vi "GagePeakHisto.vi"() -> ()   [LabVIEW 2017]
uses:
  <vilib>/measure/mamon.llb/Waveform Peak Detection for N Chan.vi
  <vilib>/Waveform/WDTOps.llb/WDT Append Waveforms DBL.vi
  <instrlib>/niHWS/nihws.llb/niHWS Store Analog Waveform DBL.vi
  <vilib>/measure/NI_MAPro.lvlib
panel:
  in  "Save waveform":bool
  in  "Save to:":path
  in  "Stop":bool
  out "Dead time (%)":dbl
  in  "Save to:":path
  in  "Save Peaks Hight":bool
  out "ChA: Histogram Peaks":dynamicdata(graph)
  in  "Peak threshold":dbl=0.5 format="%.2p"
  out "Board":string
  out "1st segment TS":string
  out "Time Interval Graph":cluster{i32[], dbl[]}(graph)
  out "Tick Frequency, Hz":u32
  in  "Trigger":T1={"Slope"=0, "Level (%)"=20, "Source"=0, "External Range"=2000, "External Coupling"=0, "External"=FALSE, "Disable"=FALSE, "External Impedance"=1} {"External Impedance" items=["50 Ohm", "HiZ"]; "External Coupling" items=["DC", "AC"]; "External Range" min=2000 max=10000 step=8000; "Slope" items=["Rising", "Falling"]; "Level (%)" min=-100 max=100; "Source" min=0 max=64 step=1}
  in  "Reset":bool
  in  "Counter source":bool
  out "Array":dbl[](array[numeric]) format="%.2f"
  out "Status":string
  in  "Channels":T2(array[cluster])=[{"Coupling"=0, "Differential Input"=FALSE, "Direct-to-ADC"=FALSE, "Range"=2000, "Impedance"=50, "DC Offset"=0, "Filter"=0}] {"Impedance" min=50 max=1000000 step=999950; "Coupling" items=["DC", "AC"]}
  in  "Acquisition":T3={"Sample Rate"=10000000.0, "Mode"=0, "Trigger Position\nin Record(%)"=50.0, "Record lenght(s)"=1.0, "Trigger Timeout(s)"=1000000.0, "Trigger Delay(s)"=0.0, "Clock mode"=enum."Internal", "Number Of Records"=10} {"Record lenght(s)" min=1.6e-05 step=1e-06 format="%.0p"; "Trigger Delay(s)" min=0.0 step=1e-06 format="%.0p"; "Trigger Position\nin Record(%)" min=0.0 step=1.0; "Mode" items=["Single", "Dual", "Quad", "Octal"]; "Sample Rate" format="%.0p"}
  in  "Length":dbl=512.0 min=0.0 step=1.0
  in  "Start Point":dbl
  out "Waveform Graph":cluster{dbl, dbl, "Data in Volts":dbl[][]}(graph) caption="Record 8  of  10"
  # "Number of records"
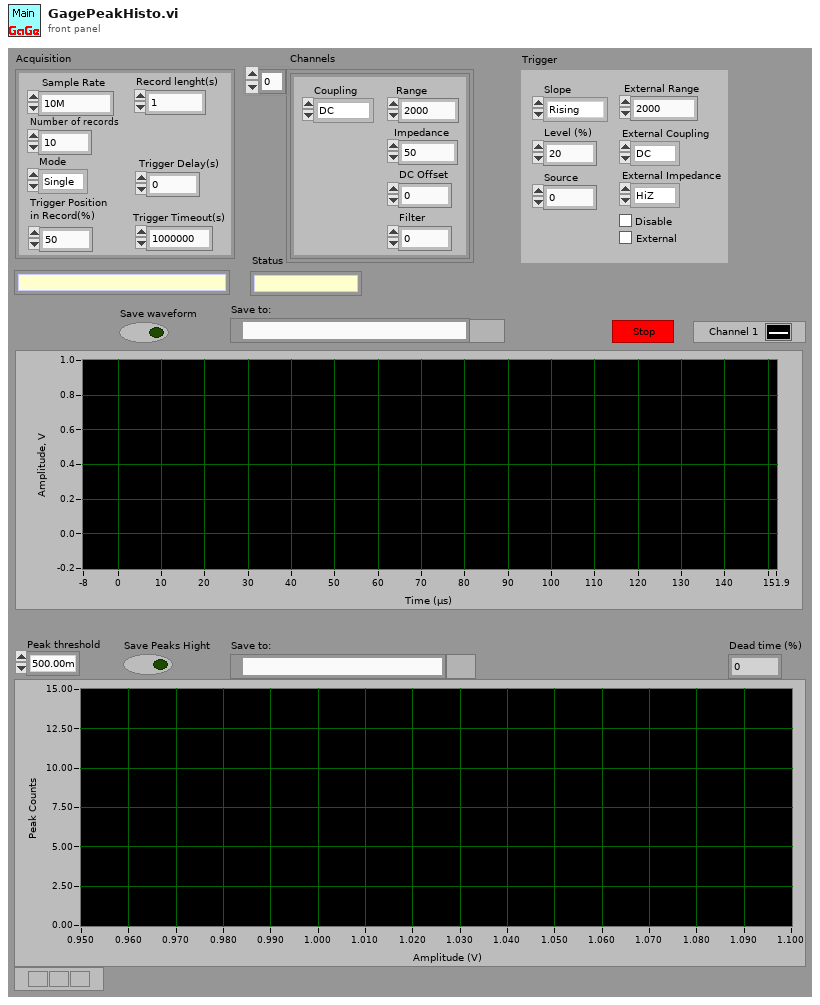
[diagram p1: front panel]
types:
  T1 = cluster{"Slope":u16, "Level (%)":i32, "Source":i32, "External Range":u32, "External Coupling":u16, "External":bool, "Disable":bool, "External Impedance":u16}
  T2 = cluster{"Coupling":u16, "Differential Input":bool, "Direct-to-ADC":bool, "Range":u32, "Impedance":u32, "DC Offset":i32, "Filter":i32}[]
  T3 = cluster{"Sample Rate":dbl, "Mode":u16, "Trigger Position\nin Record(%)":dbl, "Record lenght(s)":dbl, "Trigger Timeout(s)":dbl, "Trigger Delay(s)":dbl, "Clock mode":enum16{"Internal", "External", "Reference"}, "Number Of Records":u32}
  T4 = enum16{"big-endian, network order", "native, host order", "little-endian"}
  T5 = cluster{"Handle":u32, "Sample size":u32, "Resolution":i32, "Offset":i32, "Channels":u32, "Boards":u32}
  T6 = cluster{"Coupling":u16, "Differential Input":bool, "Direct-to-ADC":bool, "Range":u32, "Impedance":u32, "DC Offset":i32, "Filter":i32}
  T7 = cluster{string, "Differential Input":bool, "Direct-to-ADC":bool, "Range":u32, "Impedance":u32, "DC Offset":i32, u32}
  T8 = cluster{"RingText.Text":string, "Level (%)":i32, "Source":i32, "External Range":u32, "RingText.Text":string, "External":bool, "Disable":bool, "RingText.Text":string}
  T9 = cluster{"RingText.Text":string, "Level (%)":i32, "Source":i32, "External Range":u32, "RingText.Text":string, "External":bool, "Disable":bool, "RingText.Text":string}[]
  T10 = cluster{"Sample Rate":dbl, "Clock mode":enum16{"Internal", "External", "Reference"}, "RingText.Text":string, dbl, dbl, dbl, dbl, "Trigger Delay(s)":dbl}
  T11 = cluster{"Handle":u32, "Sample Size":u32, "Resolution":i32, "Offset":i32, "Channels":u32, "Boards":u32}
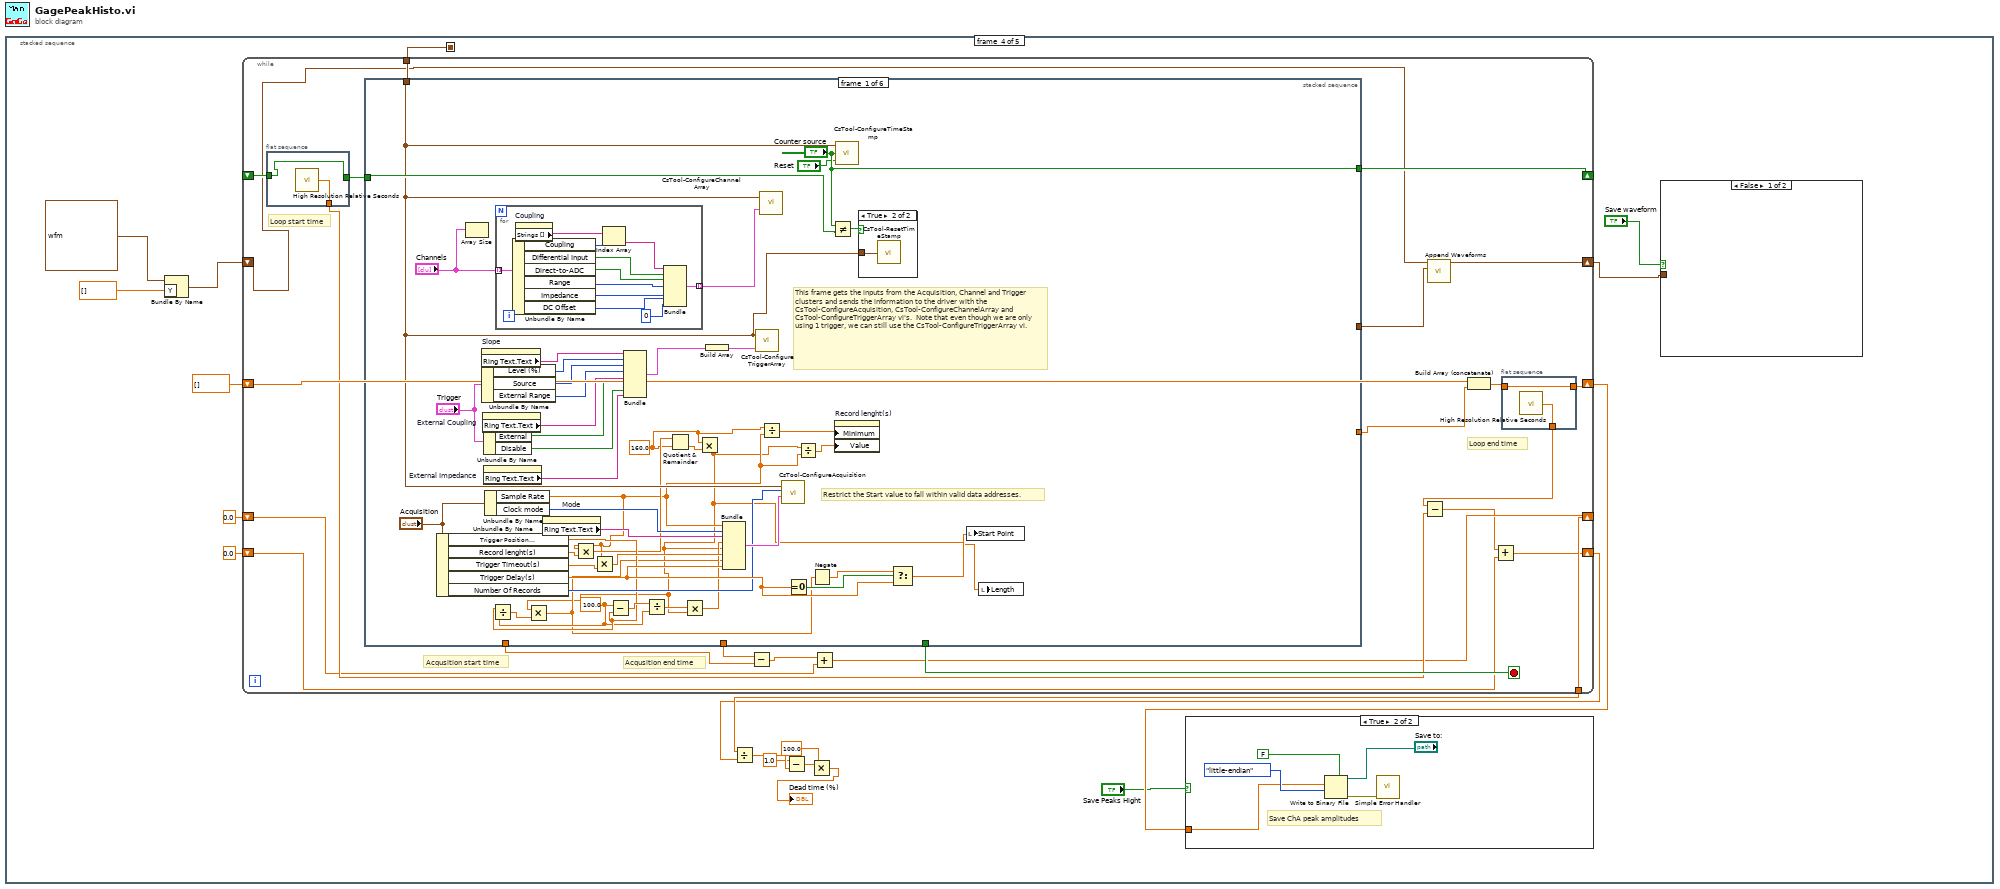
[diagram p0: block diagram]
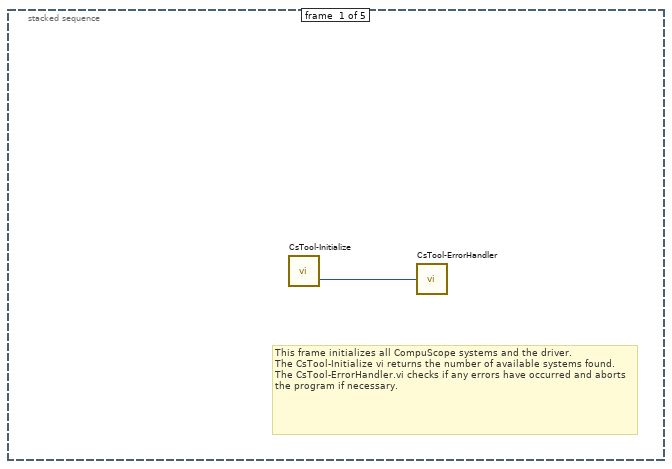
[diagram p2: hidden frame]
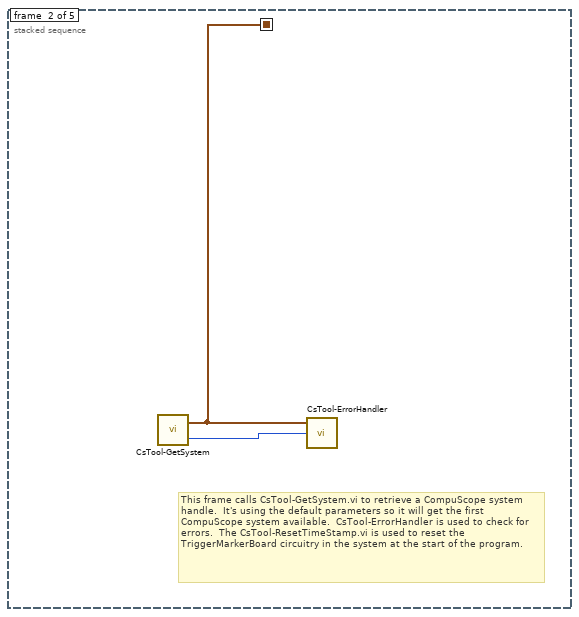
[diagram p3: hidden frame]
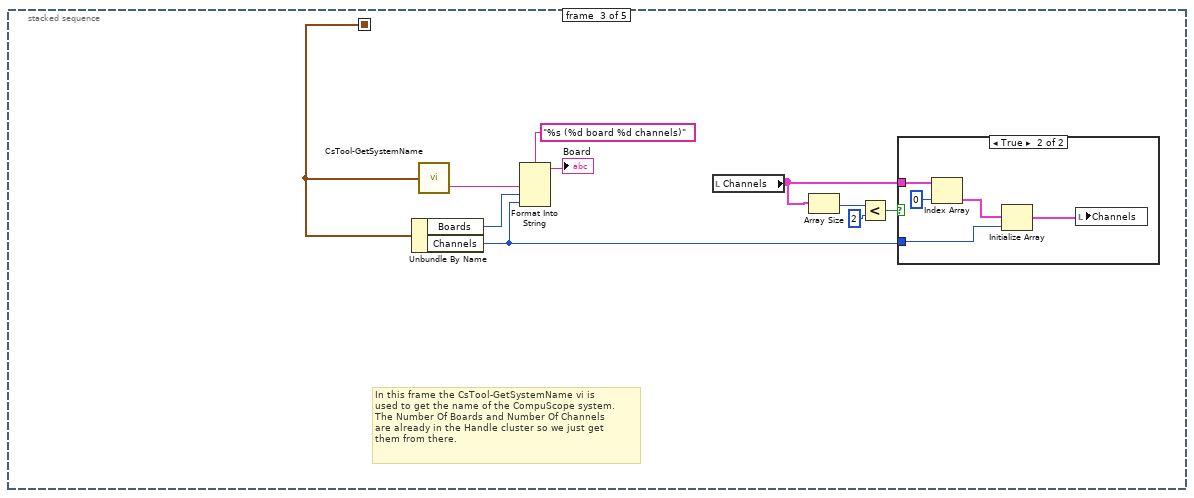
[diagram p4: hidden frame]
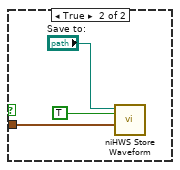
[diagram p6: hidden frame]
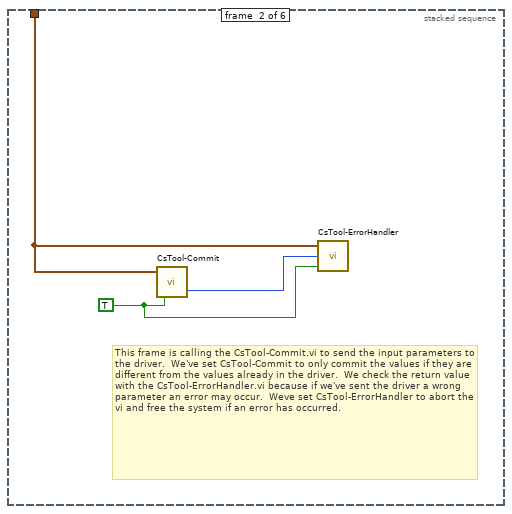
[diagram p9: hidden frame]
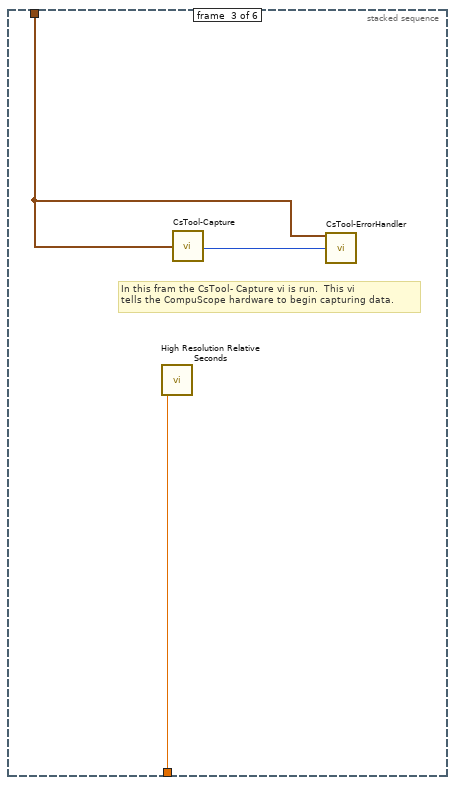
[diagram p10: hidden frame]
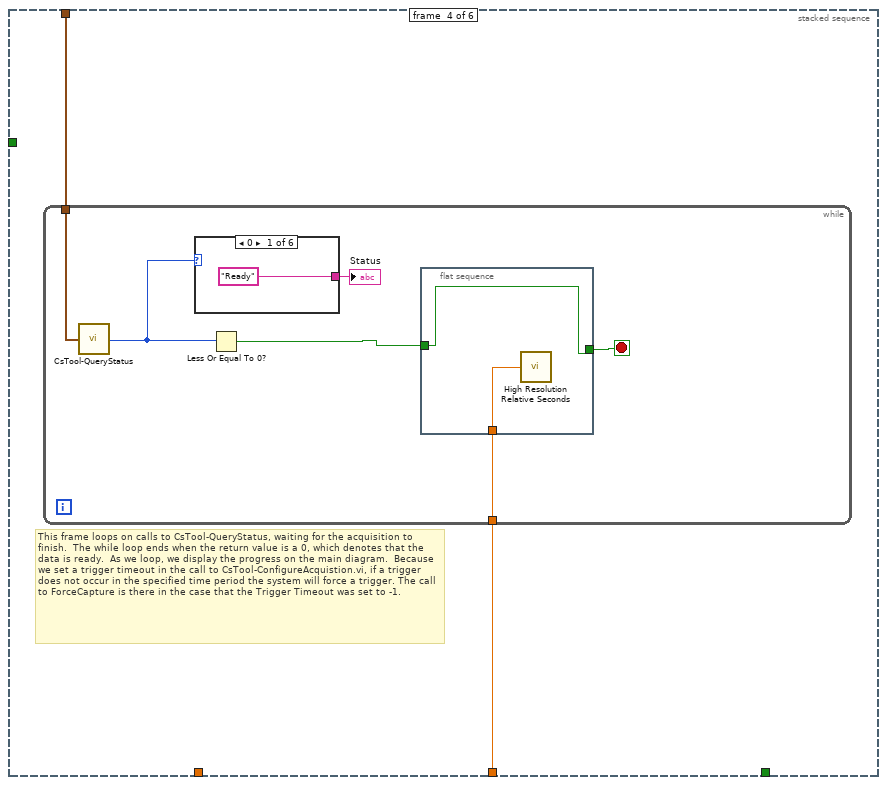
[diagram p11: hidden frame]
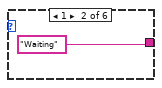
[diagram p12: hidden frame]
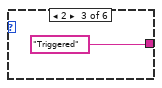
[diagram p13: hidden frame]
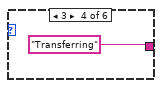
[diagram p14: hidden frame]
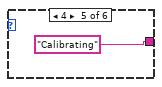
[diagram p15: hidden frame]
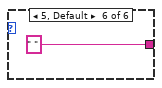
[diagram p16: hidden frame]
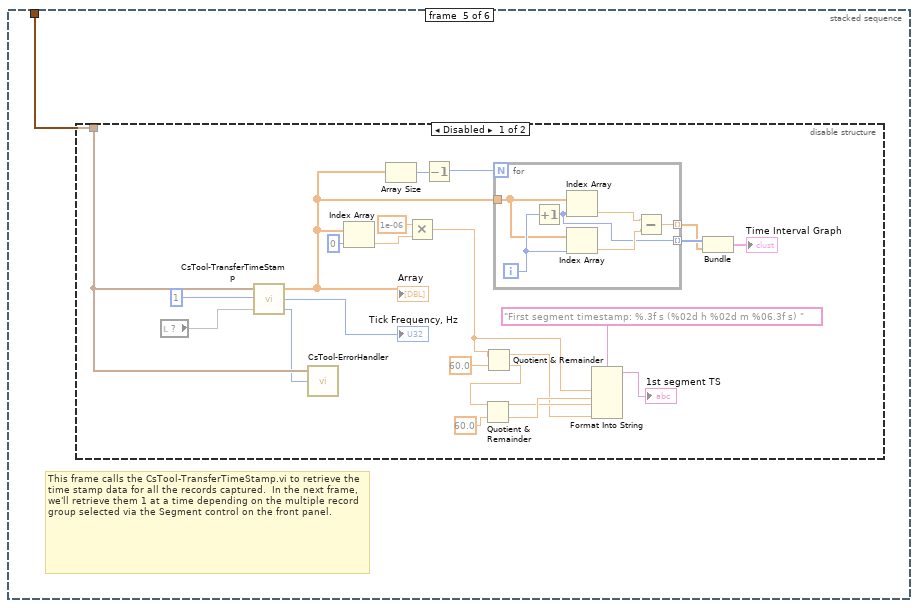
[diagram p17: hidden frame]
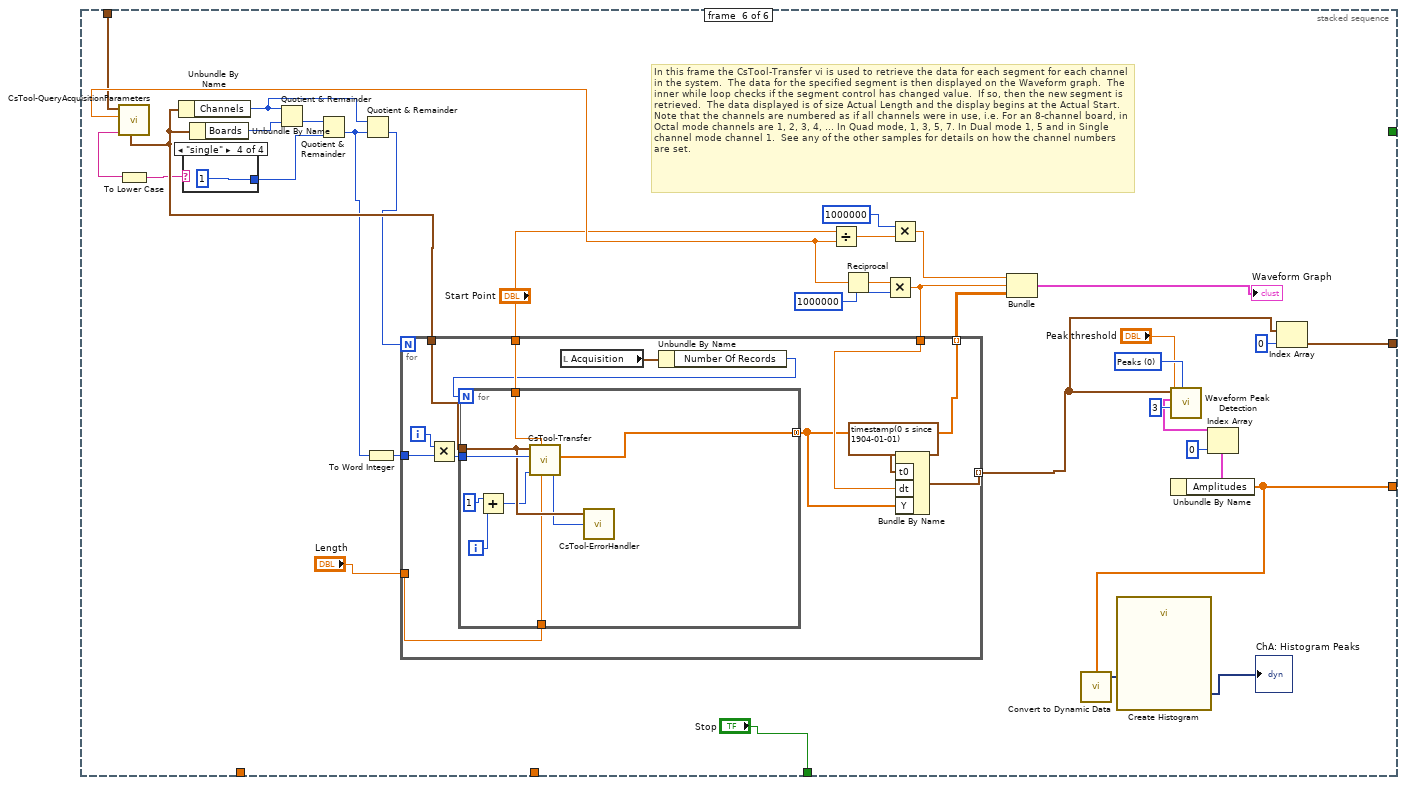
[diagram p19: hidden frame]
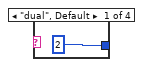
[diagram p20: hidden frame]
diagram:
  n1 = stacked-sequence {
    seq-local: [_ w2 _ _ _] -> [_ _ w13 w36 w240]
    frame #0 {
      # "This frame initializes all CompuScope systems and the driver.\nThe CsTool-Initialize vi returns the number of available systems found.  The CsTool-ErrorHandler.vi checks if any errors have occurred and aborts the program if necessary."
      n2 = call <userlib>:"CsTool-Initialize.vi"() -> ("Error Code"=w1:i32)  [unwired: 1 out]
      n3 = call <userlib>:"CsTool-ErrorHandler.vi"("Error Code"=w1) -> ()  [unwired: 2 in, 1 out]
    }
    frame #1 {
      # "This frame calls CsTool-GetSystem.vi to retrieve a CompuScope system handle.  It's using the default parameters so it will get the first CompuScope system available.  CsTool-ErrorHandler is used to check for errors.  The CsTool-ResetTimeStamp.vi is used to reset the TriggerMarkerBoard circuitry in the system at the start of the program."
      n4 = call <userlib>:"CsTool-GetSystem.vi"() -> ("Error Code"=w3:i32, "Handle Cluster"=w2:T5)  [unwired: 4 in]
      n5 = call <userlib>:"CsTool-ErrorHandler.vi"("Error Code"=w3, "Handle Cluster"=w2) -> ()  [unwired: 1 in, 1 out]
    }
    frame #2 {
      # "In this frame the CsTool-GetSystemName vi is \nused to get the name of the CompuScope system.\nThe Number Of Boards and Number Of Channels \nare already in the Handle cluster so we just get \nthem from there."
      n6 = Unbundle By Name(w13) -> ("Boards"=w5:u32, "Channels"=w6:u32)
      n7 = call <userlib>:"CsTool-GetSystemName.vi"("Handle Cluster"=w13) -> ("System Name"=w7:string)  [unwired: 1 out]
      n8 = Format Into String(format string="%s (%d board %d channels)", w7, w5, w6) -> (resulting string=→"Board":string)  [unwired: 2 in, 1 out]
      n9 = local read "Channels"() -> (w11:T2)
      n10 = Array Size(array=w11) -> (size(s)=w10:i32)
      n11 = Less?(x=w10, y=2) -> (x < y?=w12:bool)
      n12 = case shown="True" w12 {
        tunnel: w6 -> [_ w18]
        tunnel: w11 -> [_ w16]
        frame False {
        }
        frame True {
          n13 = Index Array(array=w16, index=0) -> (element=w15:T6)
          n14 = Initialize Array(w15, w18) -> (w14:T2)
          n15 = local write "Channels"(w14) -> ()
        }
      }
    }
    frame #3 {
      n16 = Bundle By Name(cluster=waveform(dbl) {"t0"=timestamp(0 s since 1904-01-01), "dt"=1.0, "Y"=[]} ("waveform"), "Y"=dbl[] []) -> (w21:waveform(dbl))
      n17 = while {
        tunnel: w36 -> [w65]
        shift-right: [w64] -> _
        shift-left: _ -> [w62]
        shift-right: [w58] -> w34
        shift-left: dbl[] [] -> [w63]
        shift-right: [w51] -> _
        shift-left: 0.0 -> [w52]
        tunnel: [w51] -> w26
        shift-right: [w49] -> w24
        shift-left: 0.0 -> [w48]
        shift-right: [w46] -> w20
        shift-left: w21 -> [w47]
        stop <- w66 stop-if-true
        # "Loop end time"
        # "Loop start time"
        # "Acqusition end time"
        # "Acqusition start time"
        n18 = flat-sequence {
          tunnel: w62 -> [w70]
          tunnel: [w70] -> w61
          tunnel: [w69] -> w56
          frame #0 {
            n19 = call <vilib>:"High Resolution Relative Seconds.vi"() -> ("relative seconds"=w69:dbl)
          }
        }
        n20 = stacked-sequence {
          tunnel: w65 -> [w93 w127 w131 w134 w149 w212]
          tunnel: [_ _ _ _ _ "Stop"] -> w66
          tunnel: ["Counter source" _ _ _ _ _] -> w64
          tunnel: w61 -> [w96 _ _ _ _ _]
          tunnel: [_ _ _ _ _ w189] -> w60
          tunnel: [_ _ w130 _ _ _] -> w54
          tunnel: [_ _ _ w133 _ _] -> w55
          tunnel: [_ _ _ _ _ w179] -> w45
          frame #0 {
            w76 = 160.0 ("y")
            w81 = 100.0 ("x")
            # "Restrict the Start value to fall within valid data addresses."
            # "This frame gets the inputs from the Acquisition, Channel and Trigger clusters and sends the information to the driver with the CsTool-ConfigureAcquisition, CsTool-ConfigureChannelArray and CsTool-ConfigureTriggerArray vi's.  Note that even though we are only using 1 trigger, we can still use the CsTool-ConfigureTriggerArray vi."
            n21 = Unbundle By Name("Acquisition") -> ("Trigger Position\nin Record(%)"=w82:dbl, "Record lenght(s)"=w88:dbl, "Trigger Timeout(s)"=w86:dbl, "Trigger Delay(s)"=w90:dbl, "Number Of Records"=w89:u32)
            n22 = Array Size(array="Channels") -> ()  [unwired: 1 out]
            n23 = property on="Slope" class="Ring (strict)"() -> ("Ring Text.Text"=w103:string)  [unwired: 2 in, 2 out]
            n24 = Unbundle By Name("Trigger") -> ("Level (%)"=w105:i32, "Source"=w107:i32, "External Range"=w108:u32)
            n25 = property on="External Coupling" class="Ring (strict)"() -> ("Ring Text.Text"=w102:string)  [unwired: 2 in, 2 out]
            n26 = property on="External Impedance" class="Ring (strict)"() -> ("Ring Text.Text"=w101:string)  [unwired: 2 in, 2 out]
            n27 = Unbundle By Name("Trigger") -> ("External"=w106:bool, "Disable"=w109:bool)
            n28 = Unbundle By Name("Acquisition") -> ("Sample Rate"=w74:dbl, "Clock mode"=w112:enum16{"Internal", "External", "Reference"})
            n29 = Divide(x=w82, y=w81) -> (x/y=w80:dbl)
            n30 = for {
              tunnel: "Channels" -> [w124] mode=indexing
              tunnel: [w125] -> w113 mode=indexing
              n31 = Unbundle By Name(w124) -> ("Coupling"=w120:u16, "Differential Input"=w126:bool, "Direct-to-ADC"=w119:bool, "Range"=w118:u32, "Impedance"=w117:u32, "DC Offset"=w116:i32)
              n32 = property on="Coupling" class="Ring (strict)"() -> ("Strings []"=w123:string[])  [unwired: 2 in, 2 out]
              n33 = Index Array(array=w123, index=w120) -> (element=w122:string)
              n34 = Bundle(w122, "Differential Input"=w126, "Direct-to-ADC"=w119, "Range"=w118, "Impedance"=w117, "DC Offset"=w116, u32 0) -> (w125:T7)  [unwired: 1 in]
            }
            n35 = property on="Mode" class="Ring (strict)"() -> ("Ring Text.Text"=w111:string)  [unwired: 2 in, 2 out]
            n36 = Multiply(x=w74, y=w88) -> (x*y=w78:dbl)
            n37 = Multiply(x=w74, y=w86) -> (x*y=w87:dbl)
            n38 = Subtract(x=w81, y=w82) -> (x-y=w84:dbl)
            n39 = Bundle("RingText.Text"=w103, "Level (%)"=w105, "Source"=w107, "External Range"=w108, "RingText.Text"=w102, "External"=w106, "Disable"=w109, "RingText.Text"=w101) -> (w100:T8)  [unwired: 1 in]
            n40 = Divide(x=w84, y=w81) -> (x/y=w85:dbl)
            n41 = Quotient & Remainder(x=w78, y=w76) -> (floor(x/y)=w77:dbl)  [unwired: 1 out]
            n42 = Multiply(x=w76, y=w77) -> (x*y=w71:dbl)
            n43 = Multiply(x=w71, y=w80) -> (x*y=w79:dbl)
            n44 = Multiply(x=w85, y=w71) -> (x*y=w83:dbl)
            n45 = Build Array(w100) -> (w99:T9)
            n46 = Bundle("Sample Rate"=w74, "Clock mode"=w112, "RingText.Text"=w111, w83, w71, w87, w79, "Trigger Delay(s)"=w90) -> (w98:T10)  [unwired: 1 in]
            n47 = call <userlib>:"CsTool-ConfigureTriggerArray.vi"("Triggers"=w99, "Handle Cluster"=w93) -> ()  [unwired: 1 out]
            n48 = call <userlib>:"CsTool-ConfigureChannelArray.vi"("Channels"=w113, "Handle Cluster"=w93) -> ()  [unwired: 1 out]
            n49 = Divide(x=w76, y=w74) -> (x/y=w75:dbl)
            n50 = call <userlib>:"CsTool-ConfigureAcquisition.vi"("Handle Cluster"=w93, "Segment Count (1)"=w89, "Acquisition"=w98) -> ()  [unwired: 2 in, 1 out]
            n51 = Equal To 0?(x=w90) -> (x = 0?=w92:bool)
            n52 = Divide(x=w71, y=w74) -> (x/y=w73:dbl)
            n53 = Negate(x=w79) -> (-x=w91:dbl)
            n54 = Not Equal?(x="Counter source", y=w96) -> (x != y?=w97:bool)
            n55 = property on="Record lenght(s)" class="DigNum (strict)"("Minimum"=w75, "Value"=w73) -> ()  [unwired: 2 in, 2 out]
            n56 = call <userlib>:"CsTool-ConfigureTimeStamp.vi"("Reset"="Reset", "Sample Clock"="Counter source", "Handle Cluster"=w93) -> ()  [unwired: 1 out]
            n57 = case shown="True" w97 {
              tunnel: w93 -> [_ w115]
              frame False {
              }
              frame True {
                n58 = call <userlib>:"CsTool-ResetTimeStamp.vi"("Handle Cluster"=w115) -> ()  [unwired: 1 out]
              }
            }
            n59 = Select(t=w91, s=w92, f=w90) -> (s? t:f=w72:dbl)
            n60 = local write "Start Point"(w72) -> ()
            n61 = local write "Length"(w71) -> ()
          }
          frame #1 {
            w128 = TRUE
            # "This frame is calling the CsTool-Commit.vi to send the input parameters to the driver.  We've set CsTool-Commit to only commit the values if they are different from the values already in the driver.  We check the return value with the CsTool-ErrorHandler.vi because if we've sent the driver a wrong parameter an error may occur.  Weve set CsTool-ErrorHandler to abort the vi and free the system if an error has occurred."
            n62 = call <userlib>:"CsTool-Commit.vi"("OnlyOnChange (t)"=w128, "Handle Cluster"=w127) -> ("Error Code"=w129:i32)  [unwired: 1 in, 1 out]
            n63 = call <userlib>:"CsTool-ErrorHandler.vi"("StopOnError (true)"=w128, "Error Code"=w129, "Handle Cluster"=w127) -> ()  [unwired: 1 out]
          }
          frame #2 {
            # "In this fram the CsTool- Capture vi is run.  This vi\ntells the CompuScope hardware to begin capturing data."
            n64 = call <vilib>:"High Resolution Relative Seconds.vi"() -> ("relative seconds"=w130:dbl)
            n65 = call <userlib>:"CsTool-Capture.vi"("Handle Cluster"=w131) -> ("Error Code"=w132:i32)
            n66 = call <userlib>:"CsTool-ErrorHandler.vi"("Error Code"=w132, "Handle Cluster"=w131) -> ()  [unwired: 1 in, 1 out]
          }
          frame #3 {
            # "This frame loops on calls to CsTool-QueryStatus, waiting for the acquisition to finish.  The while loop ends when the return value is a 0, which denotes that the data is ready.  As we loop, we display the progress on the main diagram.  Because we set a trigger timeout in the call to CsTool-ConfigureAcquistion.vi, if a trigger does not occur in the specified time period the system will force a trigger. The call to ForceCapture is there in the case that the Trigger Timeout was set to -1."
            n67 = while {
              tunnel: w134 -> [w138]
              tunnel: [w136] -> w133
              stop <- w137 stop-if-true
              n68 = call <userlib>:"CsTool-QueryStatus.vi"("Handle Cluster"=w138) -> ("Status"=w139:i32)
              n69 = case shown="0" w139 {
                tunnel: ["Ready" "Waiting" "Triggered" "Transferring" "Calibrating" " "] -> w140
                frame 0 {
                }
                frame 1 {
                }
                frame 2 {
                }
                frame 3 {
                }
                frame 4 {
                }
                frame 5, Default {
                }
              }
              "Status" <- w140
              n70 = Less Or Equal To 0?(x=w139) -> (x <= 0?=w135:bool)
              n71 = flat-sequence {
                tunnel: w135 -> [w142]
                tunnel: [w142] -> w137
                tunnel: [w141] -> w136
                frame #0 {
                  n72 = call <vilib>:"High Resolution Relative Seconds.vi"() -> ("relative seconds"=w141:dbl)
                }
              }
            }
          }
          frame #4 {
            # "This frame calls the CsTool-TransferTimeStamp.vi to retrieve the time stamp data for all the records captured.  In the next frame, we'll retrieve them 1 at a time depending on the multiple record group selected via the Segment control on the front panel."
            n73 = disable-structure shown="Disabled" {
              disable-tunnel: w149 -> [w151 _]
              frame Disabled {
                n74 = local read item#-1() -> (w171)
                n75 = call <userlib>:"CsTool-TransferTimeStamp.vi"("Length (1)"=w171, "Segment (1)"=1, "Handle Cluster"=w151) -> ("Error Code"=w150:i32, "Tick Frequency"=→"Tick Frequency, Hz":u32, "TS Time"=w167:dbl[])
                "Array" <- w167
                n76 = call <userlib>:"CsTool-ErrorHandler.vi"("Error Code"=w150, "Handle Cluster"=w151) -> ()  [unwired: 1 in, 1 out]
                n77 = Index Array(array=w167, index=0) -> (element=w165:dbl)
                n78 = Array Size(array=w167) -> (size(s)=w169:i32)
                n79 = Multiply(x=1e-06, y=w165) -> (x*y=w159:dbl)
                n80 = Decrement(x=w169) -> (x-1=w168:i32)
                n81 = Quotient & Remainder(x=w159, y=60.0) -> (x-y*floor(x/y)=w156:dbl, floor(x/y)=w162:dbl)
                n82 = Quotient & Remainder(x=w162, y=60.0) -> (x-y*floor(x/y)=w157:dbl, floor(x/y)=w158:dbl)
                n83 = for {
                  N: w168 -> [_]
                  tunnel: w167 -> [w175]
                  tunnel: [w174] -> w153 mode=indexing
                  tunnel: [w173] -> w154 mode=indexing
                  i -> [w178]
                  n84 = Increment(x=w178) -> (x+1=w173:i32)
                  n85 = Index Array(array=w175, index=w173) -> (element=w177:dbl)
                  n86 = Index Array(array=w175, index=w178) -> (element=w176:dbl)
                  n87 = Subtract(x=w177, y=w176) -> (x-y=w174:dbl)
                }
                n88 = Format Into String(format string="First segment timestamp: %.3f s (%02d h %02d m %06.3f s) ", w159, w158, w157, w156) -> (resulting string=→"1st segment TS":string)  [unwired: 2 in, 1 out]
                n89 = Bundle(w154, w153) -> (→"Time Interval Graph":cluster{i32[], dbl[]})  [unwired: 1 in]
              }
              frame Enabled {
              }
            }
          }
          frame #5 {
            w195 = u16 0 items=["Peaks", "Valleys"] ("peaks/valleys")
            # "In this frame the CsTool-Transfer vi is used to retrieve the data for each segment for each channel in the system.  The data for the specified segment is then displayed on the Waveform graph.  The inner while loop checks if the segment control has changed value.  If so, then the new segment is retrieved.  The data displayed is of size Actual Length and the display begins at the Actual Start. Note that the channels are numbered as if all channels were in use, i.e. For an 8-channel board, in Octal mode channels are 1, 2, 3, 4, ... In Quad mode, 1, 3, 5, 7. In Dual mode 1, 5 and in Single channel mode channel 1.  See any of the other samples for details on how the channel numbers are set."
            n90 = call <userlib>:"CsTool-QueryAcquisitionParameters.vi"("Handle Cluster"=w212) -> ("Output Handle Cluster"=w211:T11, "Mode"=w210:string, "Sample Rate"=w213:dbl)  [unwired: 8 out]
            n91 = To Lower Case(string=w210) -> (all lower case string=w209:string)
            n92 = Unbundle By Name(w211) -> ("Channels"=w205:u32)
            n93 = case shown="\"single\"" w209 {
              tunnel: [2 4 8 1] -> w206
              frame "dual", Default {
              }
              frame "quad" {
              }
              frame "octal" {
              }
              frame "single" {
              }
            }
            n94 = Unbundle By Name(w211) -> ("Boards"=w208:u32)
            n95 = Quotient & Remainder(x=w205, y=w208) -> (floor(x/y)=w207:u32)  [unwired: 1 out]
            n96 = Quotient & Remainder(x=w207, y=w206) -> (floor(x/y)=w204:u32)  [unwired: 1 out]
            n97 = Quotient & Remainder(x=w205, y=w204) -> (floor(x/y)=w203:u32)  [unwired: 1 out]
            n98 = To Word Integer(number=w204) -> (16bit integer=w202:i16)
            n99 = Divide(x="Start Point", y=w213) -> (x/y=w200:dbl)
            n100 = Reciprocal(x=w213) -> (1/x=w196:dbl)
            n101 = Multiply(x=w196, y=1000000) -> (x*y=w184:dbl)
            n102 = for {
              N: w203 -> [_]
              tunnel: w211 -> [w222]
              tunnel: w202 -> [w224]
              tunnel: "Start Point" -> [w221]
              tunnel: "Length" -> [w220]
              tunnel: w184 -> [w219]
              tunnel: [w218] -> w182 mode=indexing
              tunnel: [w217] -> w180 mode=indexing
              i -> [w225]
              n103 = Multiply(x=w225, y=w224) -> (x*y=w223:i32)
              n104 = local read "Acquisition"() -> (w215:T3)
              n105 = Unbundle By Name(w215) -> ("Number Of Records"=w214:u32)
              n106 = for {
                N: w214 -> [_]
                tunnel: w223 -> [w234]
                tunnel: w222 -> [w233]
                tunnel: w221 -> [w228]
                tunnel: w220 -> [w227]
                tunnel: [w226] -> w218 mode=concatenating
                i -> [w230]
                n107 = Add(x=1, y=w230) -> (x+y=w229:i32)
                n108 = call <userlib>:"CsTool-Transfer.vi"("Length (4096)"=w227, "Start (0)"=w228, "Segment (1)"=w229, "Channel (0)"=w234, "Handle Cluster"=w233) -> ("Error Code"=w232:i32, "Data in Volts"=w226:dbl[])  [unwired: 1 in, 2 out]
                n109 = call <userlib>:"CsTool-ErrorHandler.vi"("Error Code"=w232, "Handle Cluster"=w233) -> ()  [unwired: 1 in, 1 out]
              }
              n110 = Bundle By Name("t0"=timestamp(0 s since 1904-01-01), "dt"=w219, "Y"=w218) -> (w217:waveform(dbl))  [unwired: 1 in]
            }
            n111 = Multiply(x=1000000, y=w200) -> (x*y=w183:dbl)
            n112 = Bundle(w183, w184, "Data in Volts"=w182) -> (→"Waveform Graph":cluster{dbl, dbl, "Data in Volts":dbl[][]})  [unwired: 1 in]
            n113 = call-poly <vilib>:"Waveform Peak Detection.vi"("peaks/valleys"=w195, "width"=3, "threshold"="Peak threshold", "Signals In"=w180) -> ("Amplitudes"=w192:cluster{"Amplitudes":dbl[]}[])  [unwired: 3 in, 4 out]
            n114 = Index Array(array=w192, index=0) -> (element=w190:cluster{"Amplitudes":dbl[]})
            n115 = Unbundle By Name(w190) -> ("Amplitudes"=w189:dbl[])
            n116 = call "Convert to Dynamic Data"("Array"=w189) -> ("Dynamic Data Type"=w188:dynamicdata)  [unwired: 3 in]
            n117 = call "Create Histogram"("Signal"=w188) -> ("Histogram"=→"ChA: Histogram Peaks":dynamicdata)  [unwired: 9 in, 1 out]
            n118 = Index Array(array=w180, index=0) -> (element=w179:waveform(dbl))
          }
        }
        n119 = Subtract(x=w55, y=w54) -> (x-y=w53:dbl)
        n120 = Add(x=w53, y=w52) -> (x+y=w51:dbl)
        n121 = Subtract(x=w57, y=w56) -> (x-y=w50:dbl)
        n122 = call-poly <vilib>:"Append Waveforms.vi"("waveform B"=w45, "waveform A"=w47) -> ("waveform out"=w46:waveform(dbl))  [unwired: 8 in, 1 out]
        n123 = Build Array (concatenate)(w63, w60) -> (w59:dbl[])
        n124 = Add(x=w50, y=w48) -> (x+y=w49:dbl)
        n125 = flat-sequence {
          tunnel: w59 -> [w68]
          tunnel: [w68] -> w58
          tunnel: [w67] -> w57
          frame #0 {
            n126 = call <vilib>:"High Resolution Relative Seconds.vi"() -> ("relative seconds"=w67:dbl)
          }
        }
      }
      n127 = Divide(x=w26, y=w24) -> (x/y=w32:dbl)
      n128 = Subtract(x=1.0, y=w32) -> (x-y=w30:dbl)
      n129 = Multiply(x=w30, y=100.0) -> (x*y=→"Dead time (%)":dbl)
      n130 = case shown="True" "Save Peaks Hight" {
        tunnel: w34 -> [_ w42]
        frame False {
        }
        frame True {
          # "Save ChA peak amplitudes"
          n131 = Write to Binary File(file (use dialog)="Save to:", data=w42, 5:FALSE ("append to file? (new file:F)"), 9:T4."little-endian" ("byte order (0:big-endian, network order)")) -> (error out=w41:errorcluster)  [unwired: 2 in, 2 out]
          n132 = call <vilib>:"Simple Error Handler.vi"("error in (no error)"=w41) -> ()  [unwired: 4 in, 5 out]
        }
      }
      n133 = case shown="False" "Save waveform" {
        tunnel: w20 -> [_ w38]
        frame False {
        }
        frame True {
          n134 = call-poly <instrlib>:"niHWS Store Waveform.vi"("data (no data)"=w38, "overwrite existing file (F:no)"=TRUE, "file path (dialog if empty)"="Save to:") -> ()  [unwired: 7 in, 2 out]
        }
      }
    }
    frame #4 {
      # "We set the Stop button (actually it's local variable) to False here so when the vi stops the Stop button will not stay depressed."
      # "In this frame, which is reached when the Stop\nis pressed, the CompuScope system is freed by\nrunning the CsTool-FreeSystem vi.  This frees any resources\nused by the system and makes it available for another\nprogram to use."
      n135 = local write "Stop"(FALSE) -> ()
      n136 = call <userlib>:"CsTool-FreeSystem.vi"("Handle Cluster"=w240) -> ()  [unwired: 1 out]
    }
  }
